vi "Relay_Control_subTest.vi"(7 "Test Result in":T2=enum."Success", 8 "error in":errorcluster, 9 "DeviceID":T1, 10 "MicrogridID":u8, 11 "Message Enqueuer in":refnum<class "Message Enqueuer.lvclass">) -> (0 "error out":errorcluster, 1 "dup DeviceID":T1, 2 "dup MicrogridID":u8, 3 "Message Enqueuer out":refnum<class "Message Enqueuer.lvclass">, 5 "Test Result out":T2=enum."Success")   [LabVIEW 2018, in "IED Test Framework.lvlib" / "IED Test.lvclass"]
doc: "This VI tests Activate and Deactive messages as part of DER_Control."
uses:
  IED Test.lvclass
  Controls/Test Result.ctl
  <vilib>/ORNL/CSEISMIC DDS/CSEISMIC DDS Base/Data Types/Controls/DeviceID.ctl
  <vilib>/ActorFramework/Message Enqueuer/Message Enqueuer.lvclass
  <vilib>/ORNL/CSEISMIC DDS/CSEISMIC DDS Base/Data Types/Relay_Control.ctl
  <vilib>/ORNL/CSEISMIC DDS/CSEISMIC DDS Base/CSEISMIC DDS.lvclass/CSEISMIC DDS.ctl
  Relay Actor/Relay Messages/Deactivate Relay Msg/Deactivate Relay Msg.lvclass/Deactivate Relay Msg.ctl
  <vilib>/ActorFramework/Message Enqueuer/Message Enqueuer.lvclass/Message Enqueuer.ctl
  Relay Actor/Relay Messages/Activate Relay Msg/Activate Relay Msg.lvclass/Activate Relay Msg.ctl
  <vilib>/ORNL/CSEISMIC DDS/CSEISMIC DDS Base/Accessors/Write DDS Reference.vi
  <vilib>/ActorFramework/Message Enqueuer/Enqueue.vi
  <vilib>/ORNL/CSEISMIC DDS/CSEISMIC DDS Base/Accessors/Read DDS Reference.vi
  <vilib>/ORNL/CSEISMIC DDS/DDS Reader/DDS Reader.lvclass
  C:/Program Files (x86)/National Instruments/LabVIEW 2018/vi.lib/ORNL/CSEISMIC DDS/CSEISMIC DDS Base/CSEISMIC DDS.lvclass
  Relay Actor/Relay Messages/Deactivate Relay Msg/Deactivate Relay Msg.lvclass
  C:/Program Files (x86)/National Instruments/LabVIEW 2018/vi.lib/ActorFramework/Message/Message.lvclass
  Relay Actor/Relay Messages/Activate Relay Msg/Activate Relay Msg.lvclass
  <vilib>/ORNL/CSEISMIC DDS/CSEISMIC DDS Base/Error Handler.vi
  <vilib>/ActorFramework/Message Priority Queue/Priority Enqueue.vi
  <vilib>/ORNL/CSEISMIC DDS/CSEISMIC DDS Base/CSEISMIC DDS.lvclass
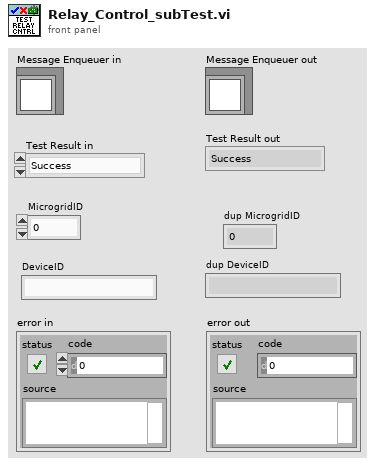
[diagram p1: front panel]
types:
  T1 = typedef "CSEISMIC DDS.lvlib/CSEISMIC DDS.lvclass/DeviceID.ctl" = string
  T2 = typedef "IED Test Framework.lvlib/IED Test.lvclass/Test Result.ctl" = enum16{"Invalid", "Success", "Failure", "Error", "Timeout"}
  T3 = typedef "CSEISMIC DDS.lvlib/CSEISMIC DDS.lvclass/Relay_Control.ctl" = cluster{"DeviceID":T1, "Activate":bool, "Deactivate":bool}
  T4 = typedef "LVDDS_library.lvlib/DDS Sample Info.ctl" = cluster{"DDS_SampleStateKind":enum32{"DDS_INVALID_SAMPLE_STATE", "DDS_READ_SAMPLE_STATE", "DDS_NOT_READ_SAMPLE_STATE"}, "DDS_ViewStateKind":enum32{"DDS_INVALID_SAMPLE_STATE", "DDS_NEW_VIEW_STATE", "DDS_NOT_NEW_VIEW_STATE"}, "DDS_InstanceStateKind":enum32{"DDS_INVALID_STATE", "DDS_ALIVE_INSTANCE_STATE", "DDS_NOT_ALIVE_DISPOSED_INSTANCE_STATE", "", "DDS_NOT_ALIVE_NO_WRITERS_INSTANCE_STATE"}, "sec":i32, "nanosec":u32, "valid_data":bool}
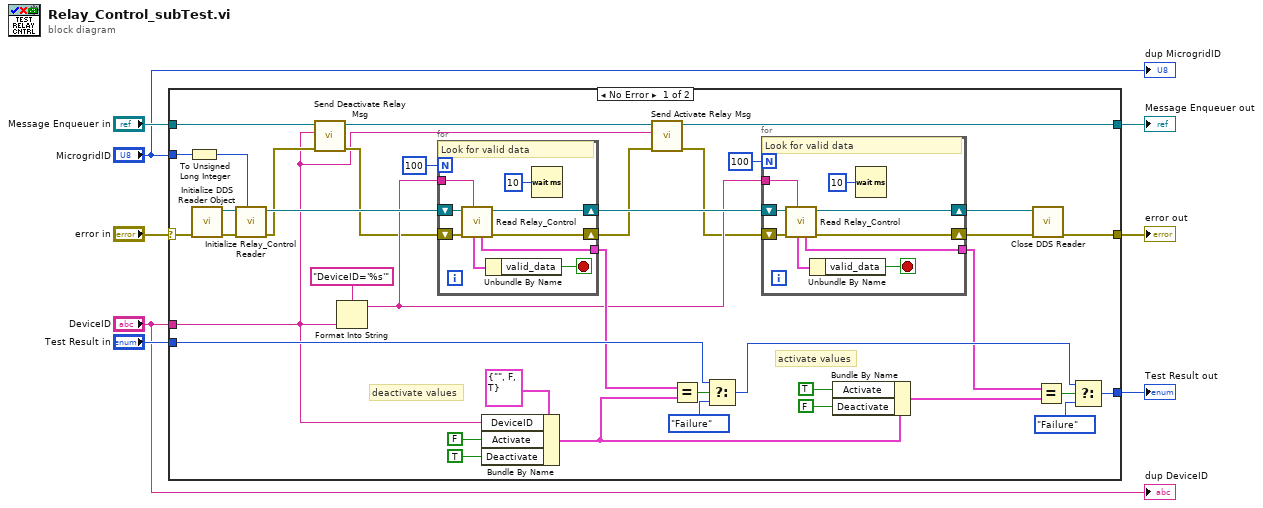
[diagram p0: block diagram]
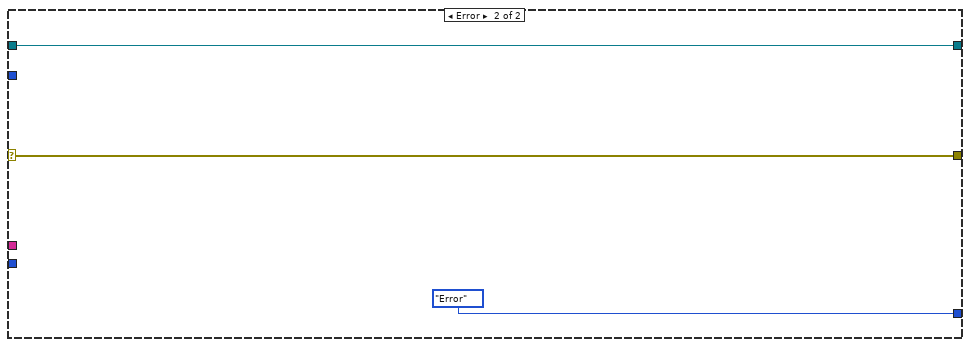
[diagram p2: hidden frame]
diagram:
  n1 = case shown="No Error" "error in" {
    selector: "error in" -> [w37 w66]
    tunnel: [w46 Test_Result."Error" ("Test Result")] -> w5
    tunnel: "DeviceID" -> [w11 _]
    tunnel: [w12 w65] -> w3
    tunnel: "MicrogridID" -> [w34 _]
    tunnel: [w31 w66] -> w4
    tunnel: "Message Enqueuer in" -> [w16 w65]
    tunnel: "Test Result in" -> [w38 _]
    frame No Error {
      # "activate values"
      # "deactivate values"
      n2 = To Unsigned Long Integer(number=w34) -> (unsigned 32bit integer=w30:u32)
      n3 = call <vilib>:"Initialize DDS Reader Object.vi"("error in"=w37) -> ("error out"=w36:errorcluster, "DDS Reader out"=w35:refnum<class "DDS Reader.lvclass">)  [unwired: 9 in]
      n4 = call <vilib>:"Initialize Relay_Control Reader.vi"("MicrogridID"=w30, "error in"=w36, "DDS Reader in"=w35) -> ("error out"=w15:errorcluster, "DDS Reader out"=w33:refnum<class "DDS Reader.lvclass">)  [unwired: 7 in]
      n5 = call "Send Deactivate Relay Msg.vi"("error in (no error)"=w15, "DeviceID"=w11, "Message Enqueuer"=w16) -> ("error out"=w14:errorcluster, "Message Enqueuer out"=w13:refnum<class "Message Enqueuer.lvclass">)  [unwired: 7 in]
      n6 = Format Into String(format string="DeviceID='%s'", w11) -> (resulting string=w22:string)  [unwired: 2 in, 1 out]
      n7 = for {
        N: 100 -> [_]
        tunnel: [w61] -> w32
        shift-right: [w63] -> w10
        shift-left: w14 -> [w64]
        shift-right: [w60] -> w26
        shift-left: w33 -> [w62]
        tunnel: w22 -> [w56]
        stop <- w57 stop-if-true
        # "Look for valid data"
        n8 = call <vilib>:"Read Relay_Control.vi"("Query condition"=w56, "error in"=w64, "DDS Reader in"=w62) -> ("error out"=w63:errorcluster, "DDS Reader out"=w60:refnum<class "DDS Reader.lvclass">, "data"=w61:T3, "DDS Sample Info"=w58:T4)  [unwired: 5 in]
        n9 = Unbundle By Name(w58) -> ("valid_data"=w57:bool)
        n10 = Wait (ms)(milliseconds to wait=u32 10) -> ()  [unwired: 1 out]
      }
      n11 = Bundle By Name(cluster=T3 {"DeviceID"="", "Activate"=FALSE, "Deactivate"=TRUE} ("Relay_Control"), "DeviceID"=w11, "Activate"=FALSE, "Deactivate"=TRUE) -> (w19:T3)
      n12 = call "Send Activate Relay Msg.vi"("error in (no error)"=w10, "DeviceID"=w11, "Message Enqueuer"=w13) -> ("error out"=w9:errorcluster, "Message Enqueuer out"=w12:refnum<class "Message Enqueuer.lvclass">)  [unwired: 7 in]
      n13 = Equal?(x=w32, y=w19) -> (x = y?=w41:bool)
      n14 = Select(t=w38, s=w41, f=Test_Result."Failure" ("Test Result")) -> (s? t:f=w45:T2)
      n15 = for {
        N: 100 -> [_]
        tunnel: [w52] -> w25
        shift-right: [w54] -> w23
        shift-left: w9 -> [w55]
        shift-right: [w51] -> w24
        shift-left: w26 -> [w53]
        tunnel: w22 -> [w47]
        stop <- w48 stop-if-true
        # "Look for valid data"
        n16 = call <vilib>:"Read Relay_Control.vi"("Query condition"=w47, "error in"=w55, "DDS Reader in"=w53) -> ("error out"=w54:errorcluster, "DDS Reader out"=w51:refnum<class "DDS Reader.lvclass">, "data"=w52:T3, "DDS Sample Info"=w49:T4)  [unwired: 5 in]
        n17 = Unbundle By Name(w49) -> ("valid_data"=w48:bool)
        n18 = Wait (ms)(milliseconds to wait=u32 10) -> ()  [unwired: 1 out]
      }
      n19 = Bundle By Name(cluster=w19, "Activate"=TRUE, "Deactivate"=FALSE) -> (w18:T3)
      n20 = call <vilib>:"Close DDS Reader.vi"("error in"=w23, "DDS Reader in"=w24) -> ("error out"=w31:errorcluster)  [unwired: 9 in]
      n21 = Equal?(x=w25, y=w18) -> (x = y?=w44:bool)
      n22 = Select(t=w45, s=w44, f=Test_Result."Failure" ("Test Result")) -> (s? t:f=w46:T2)
    }
    frame Error {
    }
  }
  "Test Result out" <- w5
  "Message Enqueuer out" <- w3
  "error out" <- w4
  "dup MicrogridID" <- "MicrogridID"
  "dup DeviceID" <- "DeviceID"
